vi "2D_array_from_string.vi"(1 "String Name":string, 2 "Show Dialog?":bool, 3 "Input string":string, 4 "Array title":string) -> (0 "2D data array":dbl[][](array[numeric]) format="%.2f")   [LabVIEW 2020]
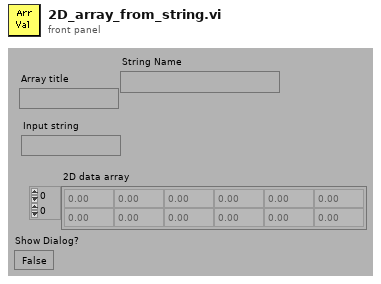
[diagram p1: front panel]
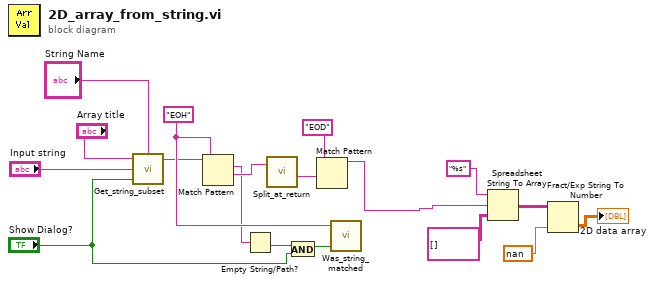
[diagram p0: block diagram]
diagram:
  w15 = "EOH"
  n1 = call "Get_string_subset.vi"("String Name"="String Name", "Show Dialog?"="Show Dialog?", "String to split"="Input string", "File Label"="Array title") -> ("Output string"=w14:string)  [unwired: 1 out]
  n2 = Match Pattern(string=w14, regular expression=w15) -> (match substring=w11:string, after substring=w18:string)  [unwired: 3 out]
  n3 = Empty String/Path?(string/path=w11) -> (empty?=w10:bool)
  n4 = call "Split_at_return.vi"("String"=w18) -> ("after substring"=w17:string)  [unwired: 1 in, 3 out]
  n5 = And(x=w10, y="Show Dialog?") -> (x .and. y?=w8:bool)
  n6 = Match Pattern(string=w17, regular expression="EOD") -> (before substring=w2:string)  [unwired: 4 out]
  n7 = call "Was_string_matched.vi"("Match Error"=w8, "Variable name"=w15) -> ()  [unwired: 1 in]
  n8 = Spreadsheet String To Array(format string="%s", spreadsheet string=w2, array type (2D Dbl)=string[][] []) -> (array=w4:string[][])  [unwired: 1 in]
  n9 = Fract/Exp String To Number(string=w4, default (0 dbl)=nan ("default (0 DBL)")) -> (number=→"2D data array":dbl[][])  [unwired: 2 in, 1 out]
